vi "清空.vi"(8 "error in (no error)":errorcluster caption="错误输入（无错误）", 11 "数据文件.lvclass":refnum<class "数据文件.lvclass">) -> (0 "error out":errorcluster caption="错误输出", 3 "数据文件.lvclass":refnum<class "数据文件.lvclass">)   [LabVIEW 2021, in "数据文件.lvclass"]
doc: "本VI是为《我和LabVIEW》一书编写的示例。\n关于本书的介绍请参考网页：\nhttp://ruanqizhen.spaces.live.com/blog/cns!5852D4F797C53FB6!4310.entry"
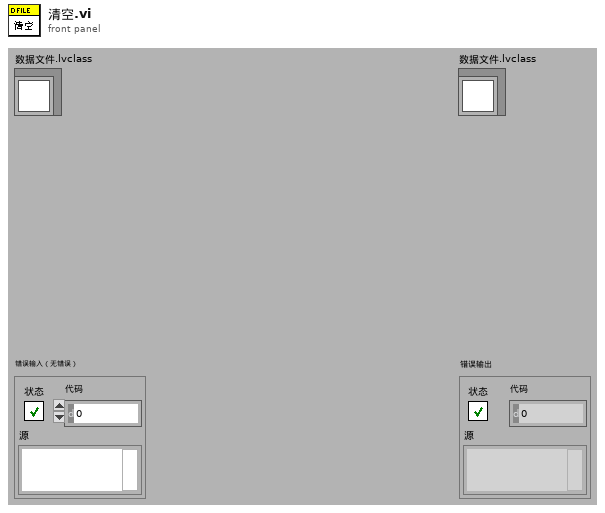
[diagram p1: front panel]
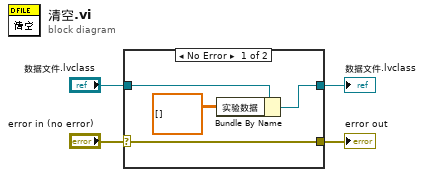
[diagram p0: block diagram]
diagram:
  n1 = case shown="No Error" "error in (no error)" {
    selector: "error in (no error)" -> [w8 w10]
    tunnel: [w8 w10] -> w3
    tunnel: [w6 w9] -> w1
    tunnel: "数据文件.lvclass" -> [w7 w9]
    frame No Error {
      n2 = Bundle By Name(cluster=w7, "实验数据"=dbl[][] []) -> (w6:refnum<class "数据文件.lvclass">)
    }
    frame Error {
    }
  }
  "error out" <- w3
  "数据文件.lvclass" <- w1
